vi "serialRead.vi"(0 "VISA resource name":refnum<visa-resource-name>="COM1", 1 "baud rate":u32=9600, 2 "data bits":u16=8 min=5 max=8 step=1, 3 "parity":u16(ring) items=["None", "Odd", "Even", "Mark", "Space"], 4 "stop bits":u16(ring)=10 items=["1.0"=10, "1.5"=15, "2.0"=20], 7 "flow control":u16(ring) items=["None"=0, "XON/XOFF"=1, "RTS/CTS"=2, "DTR/DSR"=4]) -> ()   [LabVIEW 2012]
doc: "The Basic Serial Read and Write example performs a Serial Port Read, a Serial Port Write, or a combination of these actions. The user selects the actions (read or write) on the front panel. If both are selected, the VI will write the data first, read data, and then close the VISA session that is opened to the port. This VI will wait until the specified number of bytes is received at the port. Only the number of bytes specified will be read.\n\nINSTRUCTIONS:\n1) Select the serial resource and configuration parameters (baud rate, data bits, parity, stop bits, flow control).\n2) Select the operations to be performed. \n3) Connect the serial port to your device. If no device is available, perform a loopback test by doing one of the following. Short pins 2 and 3 on a RS-232 cable or short pin 4 to pin 8 and pin 5 to pin 9 on a RS-485/422 cable. \n4) Run the VI to see the data read. (The \"read string\" will match the \"string to write\" if a loopback test was performed.)\n\nNote: The parameters set for the serial port must match the parameters of the connected instrument or device. In this example, the bytes to read parameter specifies the number of bytes that the serial port reads. If there were more bytes at the port than the number specified in bytes to read, those bytes would not be read. Also, if you specify to read more bytes than the number of bytes actually read, you might receive a timeout error message.\n\nOn the block diagram, the Configure Serial Port VI sets the configuration parameters. The front panel displays the controls used to configure the basic parameters, such as baud rate, data bits, and parity. Constants configure the other parameters the user probably does not need set. After the VISA Configure Serial Port VI opens the VISA session and configures the port, the VI passes the VISA resource name to other VIs that perform operations on that VISA resource. The VISA Write function sends a command to the serial device and the VISA Read function returns data based on the command. The VISA Close function then closes the reference to the serial device. It is important to close the reference; otherwise communication through with that port through protocols other than VISA might not be possible."
uses:
  <vilib>/Instr/_visa.llb/VISA Configure Serial Port (Instr).vi
panel:
  out "Thermometer":dbl(slide) scale=0.0..100.0
  out "Period 2":dbl(graph)
  out "Freq":dbl
  out "Period (ms)":u32
  out "Humidity":dbl(graph)
  out "Temperature":dbl(graph)
  out "Pressure":dbl(graph)
  out "Boolean array":bool[](array[boolean])
  out "element":u8
  out "Magnetometer":cluster{dbl, dbl, dbl}(graph)
  out "Gyro":cluster{dbl, dbl, dbl}(graph)
  out "Accelerometer":cluster{dbl, dbl, dbl}(graph)
  in  "stop":bool
  out "Raw Packet data (hex)":u8[](array[numeric]) format="%x"
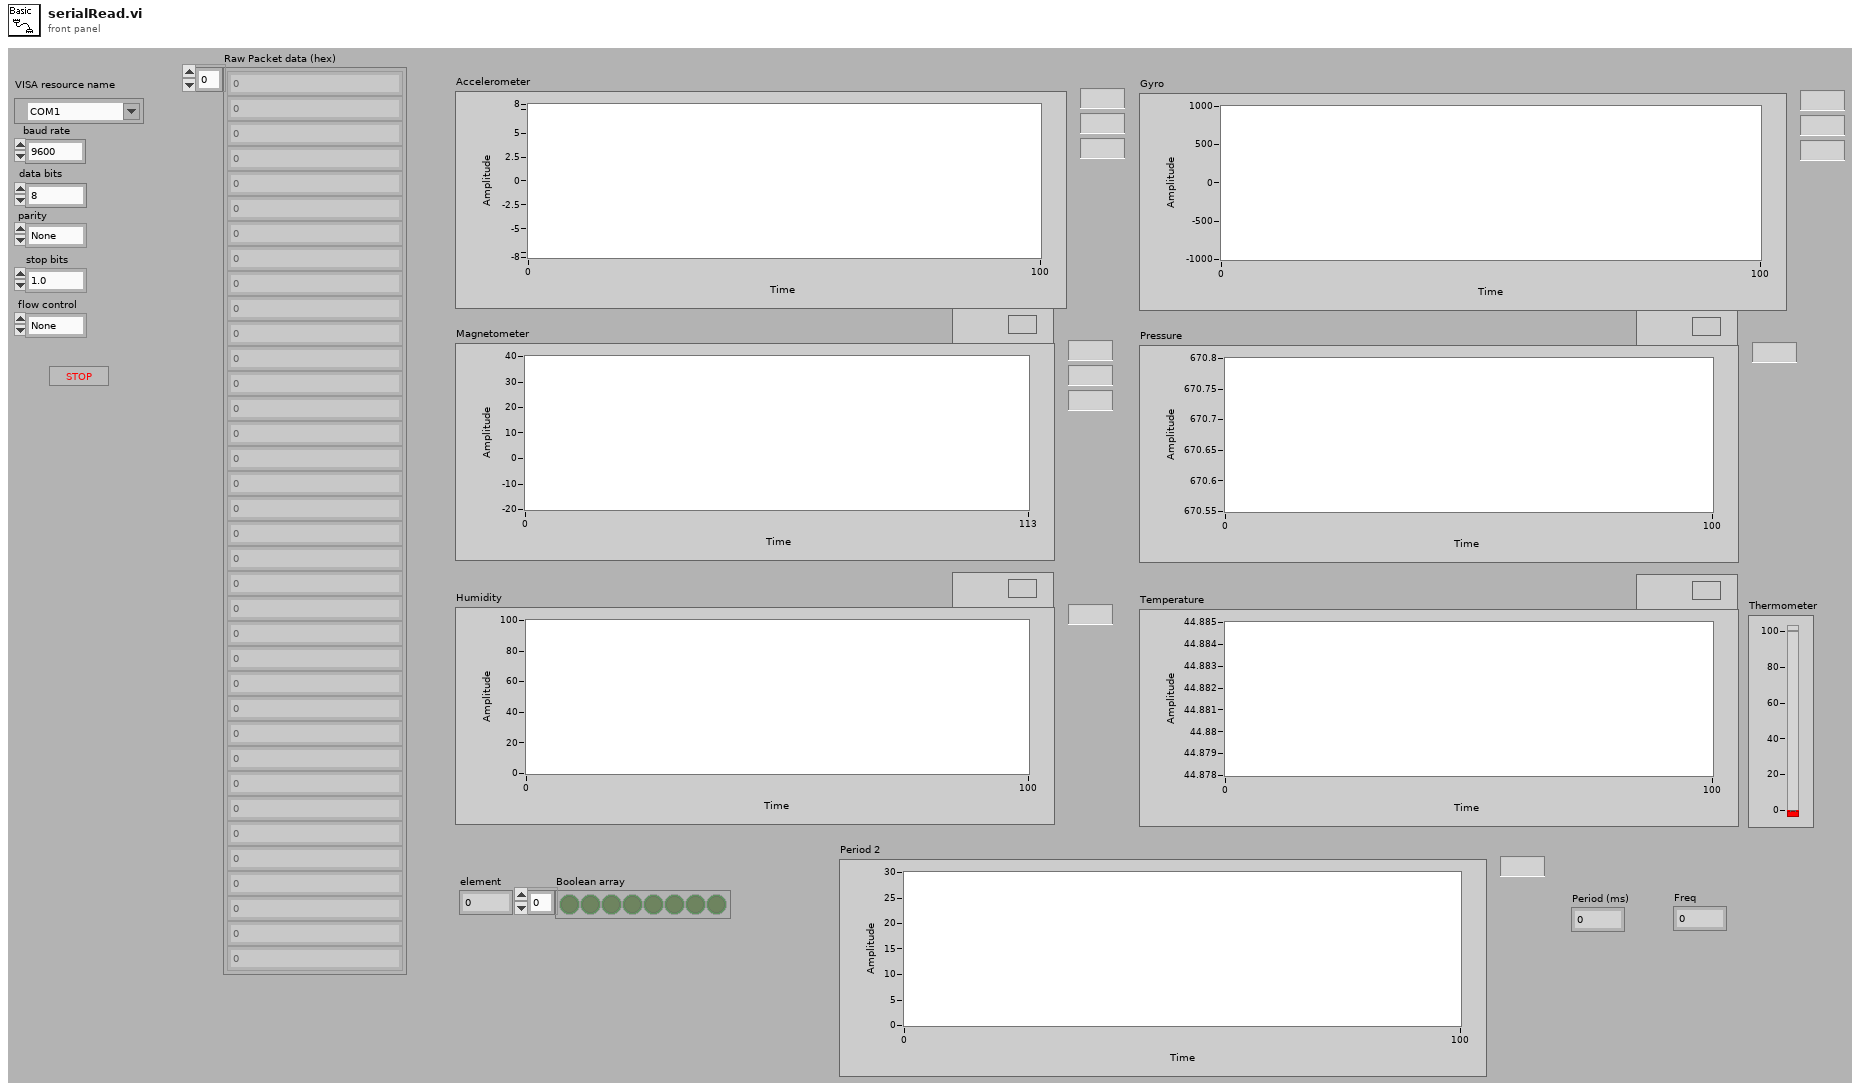
[diagram p1: front panel]
types:
  T1 = cluster{"Acceleration":dbl[], "Gyro":dbl[], "Magnetometer":dbl[], "Temperature":dbl, "Pressure":dbl, "Humidity":dbl}
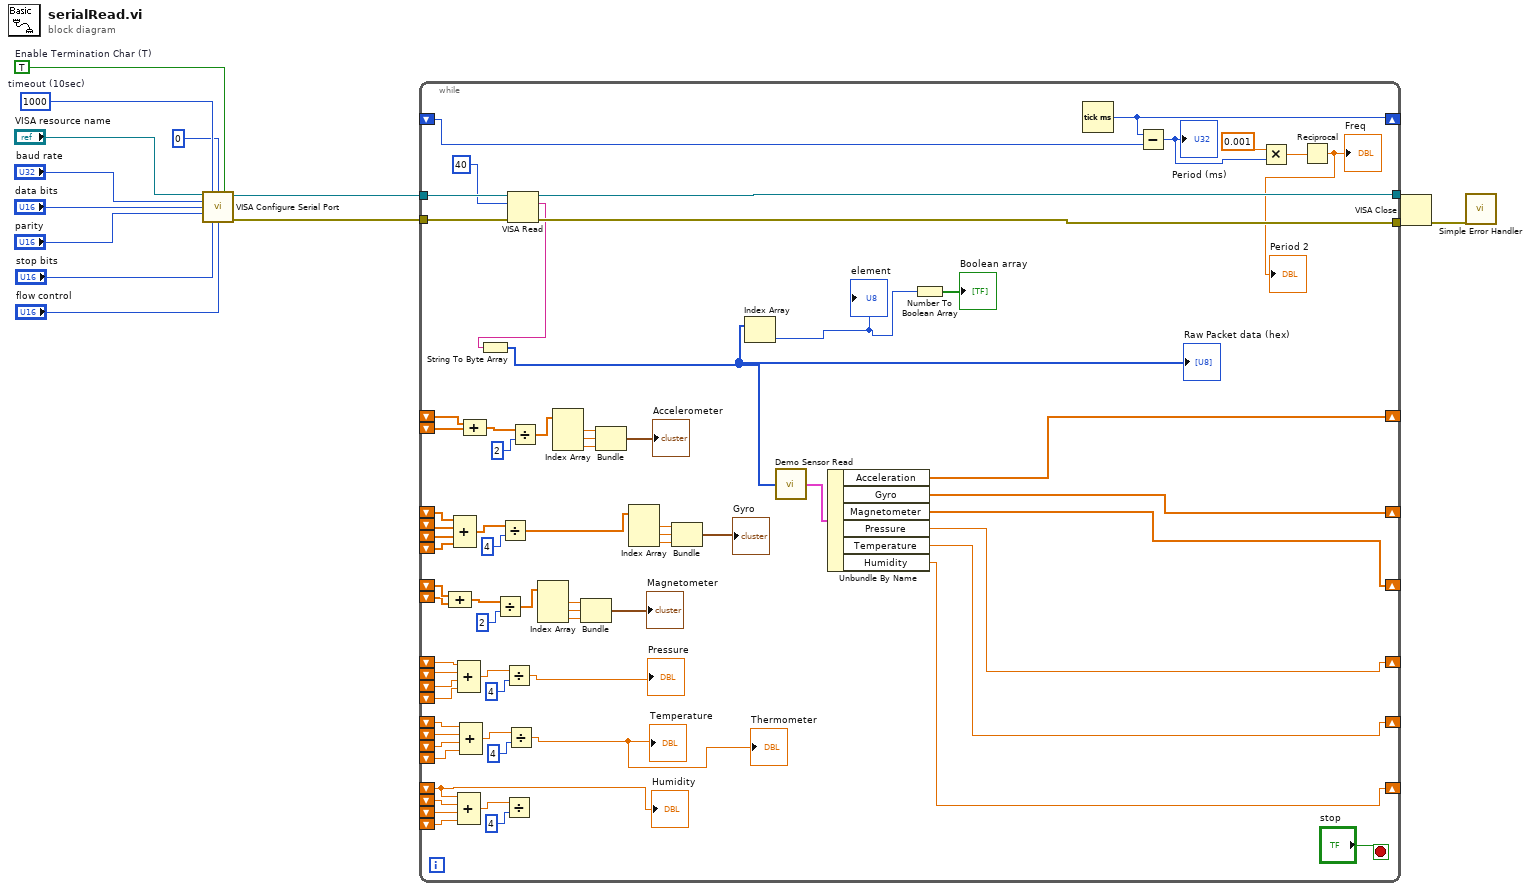
[diagram p0: block diagram]
diagram:
  w7 = TRUE  # Enable Termination Char (T)
  w8 = u32 1000  # timeout (10sec)
  n1 = call-poly "VISA Configure Serial Port"("VISA resource name"="VISA resource name", "timeout (10sec)"=w8, "termination char\n(0xA = '\\n' = LF)"=u8 0 ("termination char\n(0xA = '\\n' = LF)"), "Enable Termination\nChar (T)"=w7, "baud rate (9600)"="baud rate", "data bits (8)"="data bits", "parity (0:none)"="parity", "stop bits (10: 1 bit)"="stop bits", "flow control (0:none)"="flow control") -> ("VISA resource name out"=w3:refnum<visa-resource-name>, "error out"=w2:errorcluster)  [unwired: 5 in]
  n2 = while {
    tunnel: [w86] -> w12
    tunnel: [w85] -> w11
    tunnel: w3 -> [w84]
    tunnel: w2 -> [w83]
    shift-right: [w75] -> _
    shift-left: _ -> [w73]
    shift-left: _ -> [w74]
    shift-right: [w65] -> _
    shift-left: _ -> [w58]
    shift-left: _ -> [w57]
    shift-right: [w55] -> _
    shift-left: _ -> [w48]
    shift-left: _ -> [w47]
    shift-right: [w29] -> _
    shift-left: _ -> [w26]
    shift-right: [w28] -> _
    shift-left: _ -> [w36]
    shift-right: [w27] -> _
    shift-left: _ -> [w18]
    shift-left: _ -> [w39]
    shift-left: _ -> [w38]
    shift-left: _ -> [w37]
    shift-left: _ -> [w35]
    shift-left: _ -> [w34]
    shift-left: _ -> [w33]
    shift-left: _ -> [w32]
    shift-left: _ -> [w31]
    shift-left: _ -> [w30]
    shift-left: _ -> [w24]
    shift-left: _ -> [w23]
    shift-right: [w22] -> _
    shift-left: _ -> [w21]
    stop <- "stop" stop-if-true
    n3 = Compound Arithmetic op=ADD(w48, w47) -> (w54:dbl[])
    n4 = Compound Arithmetic op=ADD(w58, w57, w24, w23) -> (w64:dbl[])
    n5 = Compound Arithmetic op=ADD(w26, w39, w38, w37) -> (w45:dbl)
    n6 = Compound Arithmetic op=ADD(w18, w32, w31, w30) -> (w41:dbl)
    n7 = Compound Arithmetic op=ADD(w36, w35, w34, w33) -> (w43:dbl)
    n8 = Compound Arithmetic op=ADD(w73, w74) -> (w72:dbl[])
    n9 = Divide(x=w54, y=2) -> (x/y=w49:dbl[])
    n10 = Divide(x=w64, y=4) -> (x/y=w59:dbl[])
    n11 = Divide(x=w45, y=4) -> (x/y=→"Pressure":dbl)
    n12 = Divide(x=w41, y=4) -> ()  [unwired: 1 out]
    n13 = Divide(x=w43, y=4) -> (x/y=→"Temperature" →"Thermometer":dbl)
    n14 = VISA Read(VISA resource name=w84, byte count=40, error in (no error)=w83) -> (VISA resource name out=w85:refnum<visa-resource-name>, read buffer=w82:string, error out=w86:errorcluster)  [unwired: 1 out]
    n15 = String To Byte Array(string=w82) -> (unsigned byte array=w77:u8[])
    "Raw Packet data (hex)" <- w77
    n16 = Divide(x=w72, y=2) -> (x/y=w67:dbl[])
    n17 = Index Array(array=w49) -> (element #1=w52:dbl, element #2=w51:dbl, element #3=w50:dbl)  [unwired: 3 in]
    n18 = Index Array(array=w67) -> (element #1=w70:dbl, element #2=w69:dbl, element #3=w68:dbl)  [unwired: 3 in]
    n19 = Bundle(w52, w51, w50) -> (→"Magnetometer":cluster{dbl, dbl, dbl})  [unwired: 1 in]
    n20 = Bundle(w70, w69, w68) -> (→"Accelerometer":cluster{dbl, dbl, dbl})  [unwired: 1 in]
    n21 = Index Array(array=w59) -> (element #1=w62:dbl, element #2=w61:dbl, element #3=w60:dbl)  [unwired: 3 in]
    n22 = Bundle(w62, w61, w60) -> (→"Gyro":cluster{dbl, dbl, dbl})  [unwired: 1 in]
    n23 = Index Array(array=w77) -> (element=w78:u8)  [unwired: 1 in]
    "element" <- w78
    n24 = call "Demo Sensor Read.vi"("Byte array"=w77) -> ("sensor output"=w76:T1)
    n25 = Unbundle By Name(w76) -> ("Acceleration"=w75:dbl[], "Gyro"=w65:dbl[], "Magnetometer"=w55:dbl[], "Pressure"=w29:dbl, "Temperature"=w28:dbl, "Humidity"=w27:dbl)
    n26 = Number To Boolean Array(number=w78) -> (Boolean array=→"Boolean array":bool[])
    n27 = Tick Count (ms)() -> (millisecond timer value=w22:u32)
    n28 = Subtract(x=w22, y=w21) -> (x-y=w17:u32)
    "Period (ms)" <- w17
    n29 = Multiply(x=0.001, y=w17) -> (x*y=w19:dbl)
    n30 = Reciprocal(x=w19) -> (1/x=→"Freq" →"Period 2":dbl)
    "Humidity" <- w18
  }
  n31 = VISA Close(VISA resource name=w11, error in (no error)=w12) -> (error out=w10:errorcluster)
  n32 = call <vilib>:"Simple Error Handler.vi"("error in (no error)"=w10) -> ()  [unwired: 4 in, 5 out]
